vi "Example_Histogram.vi"() -> ()   [LabVIEW 2013]
uses:
  Instance           5 25Saved   Example_Histogram .vi
panel:
  out "Rate Counter\nStop Channel":i32
  out "Open Status":errorcluster
  in  "nSlot":i32=5
  in  "Start Time [ps]":i64
  out "Rate Counter\nStart Channel":i32
  in  "Bins":i32=100 min=1 max=900 step=100
  in  "BinSize":i32(ring) items=["320 ps", "640 ps", "1.28 ns", "2.56 ns", "5.12 ns", "10.24 ns", "20.48 ns", "40.96 ns", "81.92 ns", "163.84 ns"]
  in  "Stop Channel":i32=1
  in  "Start Channel":i32
  in  "nHistogram":i32
  out "Close Status":errorcluster
  in  "Stop Loop":bool
  out "histogramVector":i32[](array[numeric])
  out "HistogramPlot":cluster{i32, i16, "histogramData":u32[]}(graph)
  out "HistogramRead Status":errorcluster
  in  "Part\nNumber":string="SD-PXE-TDC-H0002"
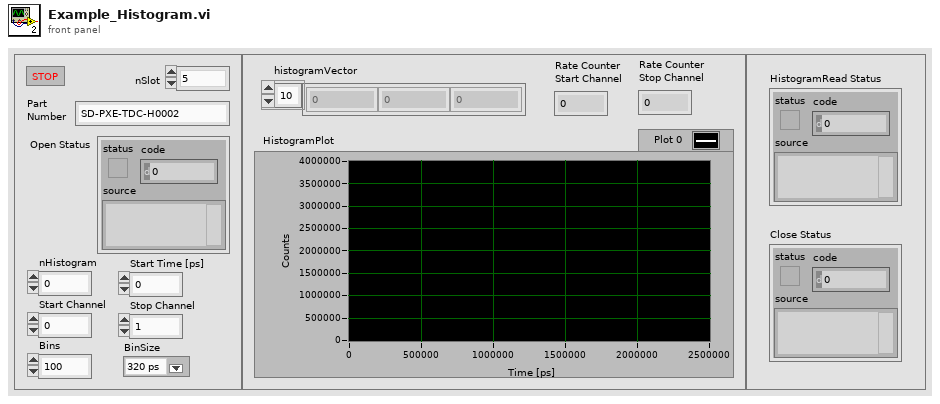
[diagram p1: front panel]
types:
  T1 = cluster{"Start Channel":i32, i16, "histogramData":u32[]}
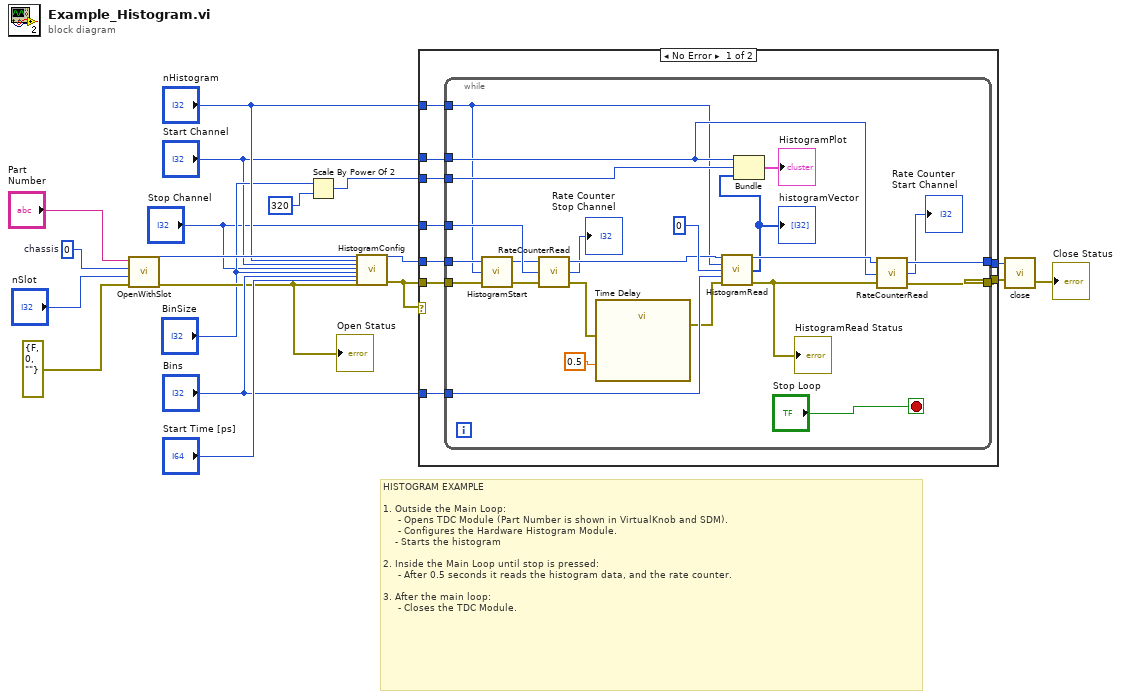
[diagram p0: block diagram]
diagram:
  w14 = 0  # chassis
  # "HISTOGRAM EXAMPLE\n\n1. Outside the Main Loop:\n     - Opens TDC Module (Part Number is shown in VirtualKnob and SDM).\n     - Configures the Hardware Histogram Module.\n    - Starts the histogram\n\n2. Inside the Main Loop until stop is pressed:\n     - After 0.5 seconds it reads the histogram data, and the rate counter.\n\n3. After the main loop:\n     - Closes the TDC Module."
  n1 = call <vilib>:"OpenWithSlot.vi"("errorIn"=errorcluster {"status"=FALSE, "code"=0, "source"=""}, "nSlot"="nSlot", "nChassis"=w14, "partNumber"="Part\nNumber") -> ("errorOut"=w11:errorcluster, "moduleID"=w17:i32)  [unwired: 2 in]
  "Open Status" <- w11
  n2 = Scale By Power Of 2(n="BinSize", x=i16 320 ("n")) -> (x*2^n=w8:i16)
  n3 = call <vilib>:"HistogramConfig.vi"("moduleID"=w17, "nHistogram"="nHistogram", "startChannel"="Start Channel", "stopChannel"="Stop Channel", "binSize"="BinSize", "nBins"="Bins", "timeOffset"="Start Time [ps]", "errorIn"=w11) -> ("moduleIDout"=w2:i32, "errorOut"=w1:errorcluster)  [unwired: 18 in]
  n4 = case shown="No Error" w1 {
    tunnel: [w28 w53] -> w5
    tunnel: [w27 w52] -> w6
    tunnel: "Bins" -> [w26 _]
    tunnel: w1 -> [w25 w52]
    tunnel: w2 -> [w24 _]
    tunnel: "nHistogram" -> [w23 w53]
    tunnel: "Start Channel" -> [w22 _]
    tunnel: w8 -> [w21 _]
    tunnel: "Stop Channel" -> [w20 _]
    frame No Error {
      n5 = while {
        tunnel: [w47] -> w28
        tunnel: [w48] -> w27
        tunnel: w23 -> [w29]
        tunnel: w26 -> [w46]
        tunnel: w25 -> [w32]
        tunnel: w24 -> [w33]
        tunnel: w22 -> [w38]
        tunnel: w21 -> [w41]
        tunnel: w20 -> [w35]
        stop <- "Stop Loop" stop-if-true
        n6 = call <vilib>:"HistogramStart.vi"("errorIn"=w32, "nHistogram"=w29, "moduleID"=w33) -> ("errorOut"=w31:errorcluster, "moduleIDout"=w30:i32)  [unwired: 1 in]
        n7 = call <vilib>:"RateCounterRead.vi"("errorIn"=w31, "nChannel"=w35, "moduleID"=w30) -> ("errorOut"=w36:errorcluster, "countRate"=→"Rate Counter\nStop Channel":i32, "moduleIDout"=w37:i32)
        n8 = call "Time Delay"("error in (no error)"=w36, "Delay Time (s)"=0.5) -> ("error out"=w42:errorcluster)  [unwired: 9 in]
        n9 = call <vilib>:"HistogramRead.vi"("moduleID"=w37, "nHistogram"=w29, "startBin"=0, "nBins"=w46, "errorIn"=w42) -> ("moduleIDout"=w45:i32, "histogramData"=w39:u32[], "errorOut"=w44:errorcluster)  [unwired: 8 in]
        "histogramVector" <- w39
        "HistogramRead Status" <- w44
        n10 = Bundle("Start Channel"=w38, w41, "histogramData"=w39) -> (→"HistogramPlot":T1)  [unwired: 1 in]
        n11 = call <vilib>:"RateCounterRead.vi"("errorIn"=w44, "nChannel"=w38, "moduleID"=w45) -> ("errorOut"=w48:errorcluster, "countRate"=→"Rate Counter\nStart Channel":i32, "moduleIDout"=w47:i32)
      }
    }
    frame Error {
    }
  }
  n12 = call <vilib>:"close.vi"("errorIn"=w6, "moduleID"=w5) -> ("errorOut"=→"Close Status":errorcluster)  [unwired: 1 in]
